vi "Initialize.vi"(8 "error in (no error)":errorcluster, 9 "Reset (True)":bool=TRUE, 10 "ID Query (True)":bool=TRUE, 11 "VISA resource name":refnum<visa-resource-name>) -> (0 "error out":errorcluster, 3 "VISA resource name out":refnum<visa-resource-name>)   [LabVIEW 2022 SP3, in "Agilent N934X Series.lvlib"]
doc: "Establishes communication with the instrument and optionally performs an instrument identification query and/or an instrument reset. It also places the instrument in a default state needed for other instrument driver operations. Therefore, call this VI before calling other instrument driver VIs for this instrument. Generally, you need to call the Initialize VI only once at the beginning of an application."
uses:
  <instrlib>/Agilent N934X Series/Agilent N934X Series.lvlib
  <vilib>/regexp/Match Regular Expression.xnode
panel:
  # "(c) 2012 - 2025 National Instruments.  ALL RIGHTS RESERVED."
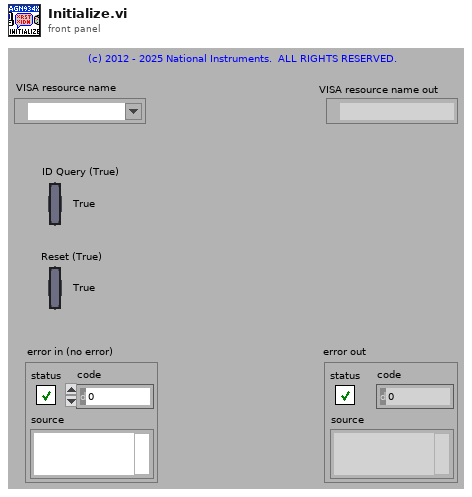
[diagram p1: front panel]
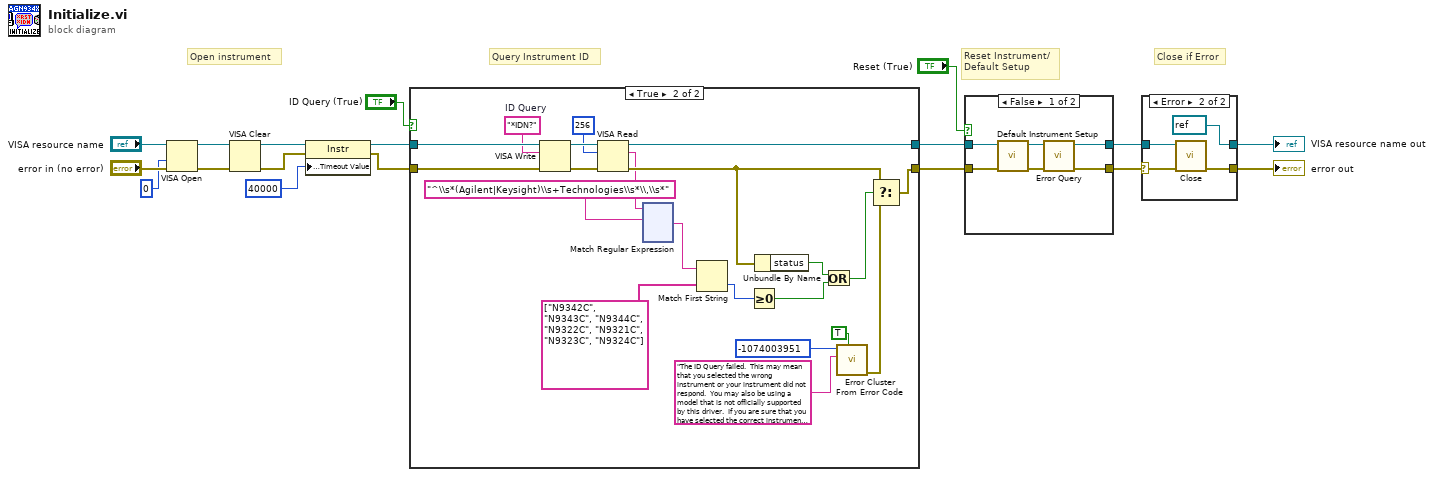
[diagram p0: block diagram]
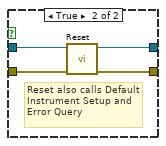
[diagram p3: hidden frame]
diagram:
  # "Close if Error"
  # "Query Instrument ID"
  # "Reset Instrument/\nDefault Setup"
  # "Open instrument"
  n1 = VISA Open(access mode=u32 0, error in (no error)="error in (no error)", VISA resource name="VISA resource name") -> (VISA resource name=w11:refnum<visa-resource-name>, error out=w10:errorcluster)  [unwired: 2 in]
  n2 = VISA Clear(VISA resource name=w11, error in (no error)=w10) -> (VISA resource name out=w9:refnum<visa-resource-name>, error out=w8:errorcluster)
  n3 = property class="Instr"(reference=w9, error in=w8, "General Settings:Timeout Value"=u32 40000) -> (reference out=w3:refnum<visa-resource-name>, error out=w2:errorcluster)
  n4 = case shown="True" "ID Query (True)" {
    tunnel: [w19 w41] -> w17
    tunnel: [w20 w38] -> w18
    tunnel: w3 -> [w20 w39]
    tunnel: w2 -> [w19 w40]
    frame False {
    }
    frame True {
      w34 = "*IDN?"  # ID Query
      n5 = VISA Write(VISA resource name=w39, write buffer=w34, error in (no error)=w40) -> (VISA resource name out=w37:refnum<visa-resource-name>, error out=w36:errorcluster)  [unwired: 1 out]
      n6 = VISA Read(VISA resource name=w37, byte count=u32 256, error in (no error)=w36) -> (VISA resource name out=w38:refnum<visa-resource-name>, read buffer=w21:string, error out=w29:errorcluster)  [unwired: 1 out]
      n7 = xnode "Match Regular Expression"("input string"=w21, "regular expression"="^\\s*(Agilent|Keysight)\\s+Technologies\\s*\\,\\s*" ("Company Name Regular Expression")) -> ("after match"=w23:string)  [unwired: 4 in, 4 out]
      n8 = Match First String(2:string[] ["N9342C", "N9343C", "N9344C", "N9322C", "N9321C", "N9323C", "N9324C"], 3:w23) -> (0:w24:i32)  [unwired: 1 out]
      n9 = Greater Or Equal To 0?(x=w24) -> (x >= 0?=w27:bool)
      n10 = Unbundle By Name(w29) -> ("status"=w28:bool)
      n11 = Or(x=w28, y=w27) -> (x .or. y?=w26:bool)
      n12 = call <vilib>:"Error Cluster From Error Code.vi"("show call chain? (False)"=TRUE, "error message (\"\")"="The ID Query failed.  This may mean that you selected the wrong instrument or your instrument did not respond.  You may also be using a model that is not officially supported by this driver.  If you are sure that you have selected the correct instrument and it is responding, try disabling the ID Query." ("Source (VI Name)"), "error code (0)"=-1074003951 ("Code")) -> ("error out"=w33:errorcluster)  [unwired: 6 in]
      n13 = Select(t=w29, s=w26, f=w33) -> (s? t:f=w41:errorcluster)
    }
  }
  n14 = case shown="False" "Reset (True)" {
    tunnel: w17 -> [w163 w165]
    tunnel: [w160 w168] -> w4
    tunnel: w18 -> [w164 w166]
    tunnel: [w161 w167] -> w5
    frame False {
      n15 = call <instrlib>:"Default Instrument Setup.vi"("error in (no error)"=w163, "VISA resource name"=w164) -> ("error out"=w159:errorcluster, "VISA resource name out"=w162:refnum<visa-resource-name>)  [unwired: 8 in]
      n16 = call <instrlib>:"Error Query.vi"("error in (no error)"=w159, "VISA resource name"=w162) -> ("error out"=w160:errorcluster, "VISA resource name out"=w161:refnum<visa-resource-name>)  [unwired: 6 in, 2 out]
    }
    frame True {
      # "Reset also calls Default Instrument Setup and Error Query"
      n17 = call <instrlib>:"Reset.vi"("error in (no error)"=w165, "VISA resource name"=w166) -> ("error out"=w168:errorcluster, "VISA resource name out"=w167:refnum<visa-resource-name>)  [unwired: 8 in]
    }
  }
  n18 = case shown="Error" w4 {
    selector: w4 -> [w169 w172]
    tunnel: w5 -> [w170 w173]
    tunnel: [w170 refnum<visa-resource-name> refnum ("VISA resource name out")] -> w7
    tunnel: [w169 w174] -> w6
    frame No Error {
    }
    frame Error {
      n19 = call <instrlib>:"Close.vi"("error in (no error)"=w172, "VISA resource name"=w173) -> ("error out"=w174:errorcluster)  [unwired: 9 in]
    }
  }
  "VISA resource name out" <- w7
  "error out" <- w6
